vi "Remove Entity.vi"(8 "error in (no error)":errorcluster, 10 "Conditum:Entity":refnum<class "Entity.lvclass">, 11 "Entity Collection in":refnum<class "Entity Collection.lvclass">) -> (0 "error out":errorcluster, 3 "Entity Collection out":refnum<class "Entity Collection.lvclass">)   [LabVIEW 2020, in "Conditum.lvlib" / "Columns.lvlib" / "Entity Collection.lvclass"]
uses:
  Entity Collection.lvclass
  Conditum-Example/User/User.lvclass
  C:/dev/lv/illuminated-g/lv-conditum/Conditum/Entity/Entity.lvclass
  C:/dev/lv/illuminated-g/lv-conditum/Conditum-Example/User/User.lvclass
  Entity/Entity.lvclass
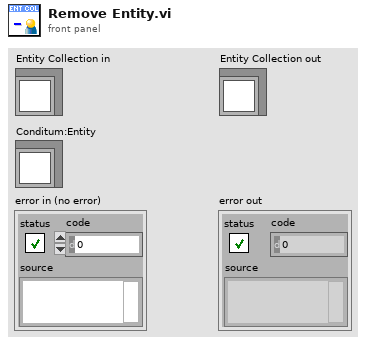
[diagram p1: front panel]
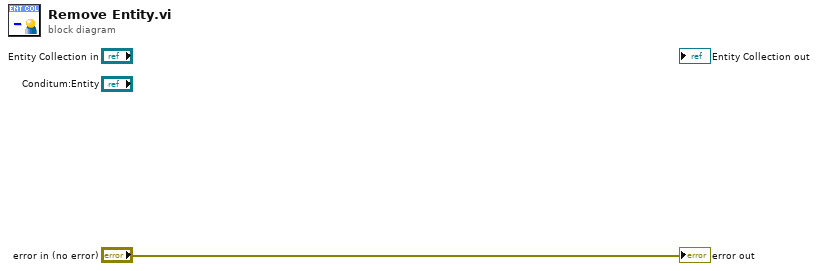
[diagram p0: block diagram]
diagram:
  "error out" <- "error in (no error)"
